vi "FT10_M4X Tester 2.vi"() -> ()   [LabVIEW 2024]
uses:
  Controls/QMH Fundamentals - Message Cluster.ctl
  <vilib>/FPGAPlugInAG/PXI-7854R/niLvFpga_Open_PXI-7854R.vi
  <vilib>/rvi/interface/common/dynamic/niFpgaDynamicAddResources.vi
  <vilib>/Utility/error.llb/Error Cluster From Error Code.vi
  <vilib>/rvi/errors/niLvFpgaAdjustHostInterfaceError.vi
  <vilib>/FPGAPlugInAG/Dynamic/niLvFpga_Close_Dynamic.vi
  <vilib>/rvi/interface/nirviOpenFPGA/nirviOpenFPGA.xnode
  FPGA Bitfiles/11_12_2024_FT10_FPGA_7854R_Main_Rev3 BitFile.lvbitx
  <vilib>/rvi/interface/nirviReadWriteControl/nirviReadWriteControl.xnode
  <vilib>/rvi/interface/nirviCloseFPGA/nirviCloseFPGA.xnode
  spcm_win32.dll
  NiFpgaLv.dll
  <vilib>/rvi/interface/Simulation/niFpgaSimulationCallBeginRW.vi
panel:
  in  "Conn2 - 75kHz":bool=TRUE
  in  "Conn2 - uSec Off":u16=6
  in  "Conn2 - uSec On":u16=7
  in  "Conn1/DIO_0_7 In":bool[](array[boolean])=[FALSE, FALSE, FALSE, FALSE, FALSE, FALSE, FALSE, FALSE]
  in  "Conn1/DIO_8_15 In":bool[](array[boolean])=[FALSE, FALSE, FALSE, FALSE, FALSE, FALSE, FALSE, FALSE]
  out "Conn1/DIO_0_7 Out":bool[](array[boolean])
  out "Conn1/DIO_8_15 Out":bool[](array[boolean])
  out "Conn1/DIO_16_23 Out":bool[](array[boolean])
  in  "Conn1/DIO_16_23 In":bool[](array[boolean])=[FALSE, FALSE, FALSE, FALSE, FALSE, FALSE, FALSE, FALSE]
  out "error out 2":errorcluster
  out "error out":errorcluster
  in  "Conn1 - uSec On":u16=7
  in  "Conn1 - uSec Off":u16=6
  in  "Conn1 - 75kHz":bool=TRUE
  in  "Conn2/DIO_0_7 In":bool[](array[boolean])=[FALSE, FALSE, FALSE, FALSE, FALSE, FALSE, FALSE, FALSE]
  in  "Conn2/DIO_8_15 In":bool[](array[boolean])=[FALSE, FALSE, FALSE, FALSE, FALSE, FALSE, FALSE, FALSE]
  out "Conn2/DIO_0_7 Out":bool[](array[boolean])
  out "Conn2/DIO_8_15 Out":bool[](array[boolean])
  out "Conn2/DIO_16_23 Out":bool[](array[boolean])
  in  "Conn2/DIO_16_23 In":bool[](array[boolean])=[FALSE, FALSE, FALSE, FALSE, FALSE, FALSE, FALSE, FALSE]
  out "Array":T1(array[cluster])
  out "Waveform Array":waveform(dbl)[](graph)
  in  "stop":bool
  in  "Read":bool
  # "Conn1/DIO_0_7"
  # "Conn1/DIO_8_15"
  # "Conn1/DIO_16_23"
  # "Conn2/DIO_0_7"
  # "Conn2/DIO_8_15"
  # "Conn2/DIO_16_23"
  # "INPUTS"
  # "OUTPUTS"
  # "INPUTS"
  # "OUTPUTS"
  # "INPUTS"
  # "OUTPUTS"
  # "INPUTS"
  # "OUTPUTS"
  # "INPUTS"
  # "OUTPUTS"
  # "INPUTS"
  # "OUTPUTS"
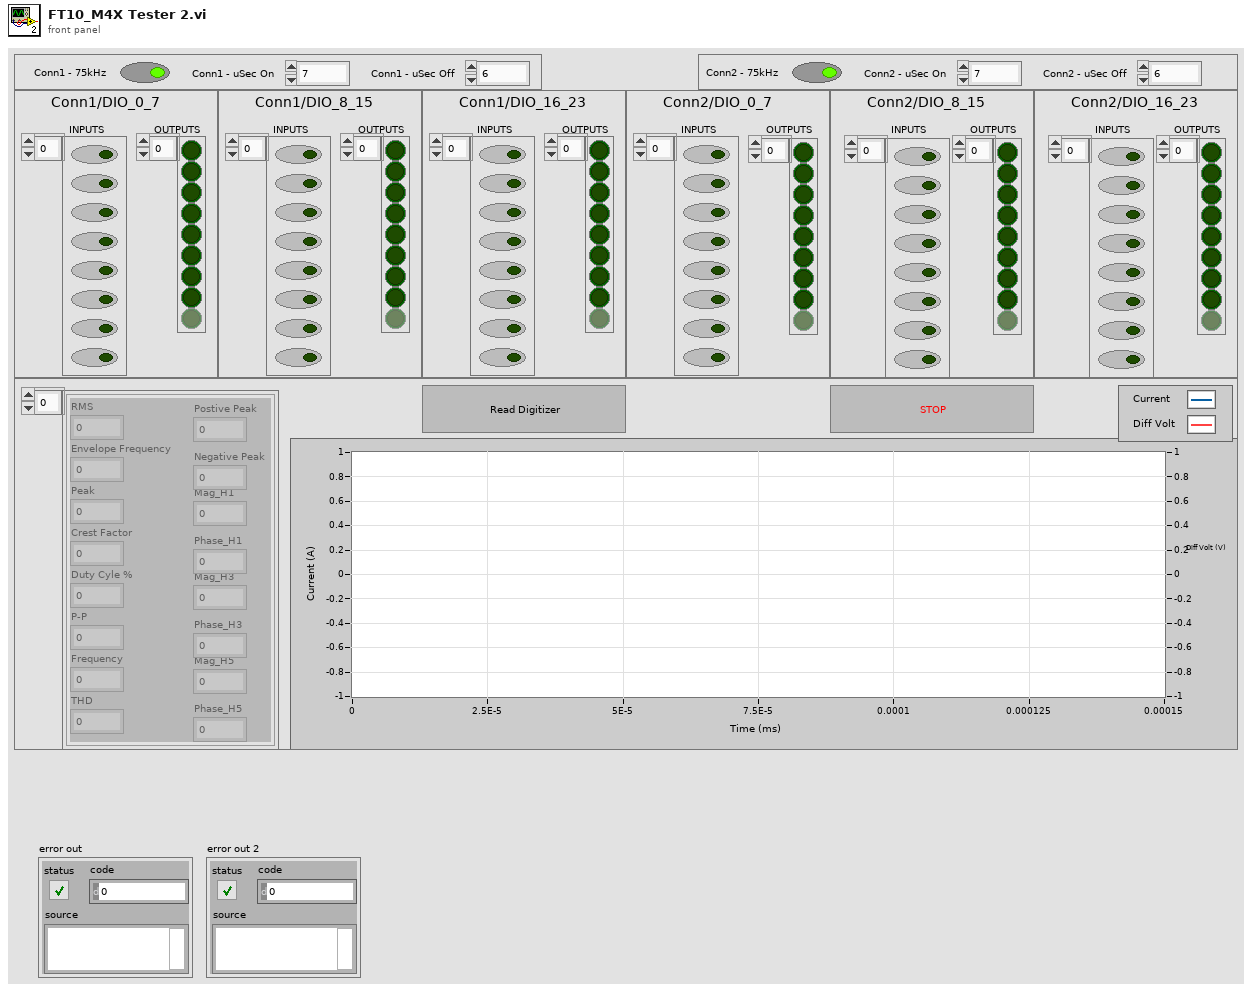
[diagram p1: front panel]
types:
  T1 = cluster{"RMS":dbl, "Envelope Frequency":dbl, "Peak":dbl, "Crest Factor":dbl, "Duty Cyle %":dbl, "P-P":dbl, "Frequency":dbl, "THD":dbl, "Postive Peak":dbl, "Negative Peak":dbl, "Mag_H1":dbl, "Phase_H1":dbl, "Mag_H3":dbl, "Phase_H3":dbl, "Mag_H5":dbl, "Phase_H5":dbl}[]
  T2 = typedef "QMH Fundamentals - Message Cluster.ctl" = cluster{"Message":string, "Message Data":variant}
  T3 = cluster{"RMS":dbl, "Envelope Frequency":dbl, "Peak":dbl, "Crest Factor":dbl, "Duty Cyle %":dbl, "P-P":dbl, "Frequency":dbl, "THD":dbl, "Postive Peak":dbl, "Negative Peak":dbl, "Mag_H1":dbl, "Phase_H1":dbl, "Mag_H3":dbl, "Phase_H3":dbl, "Mag_H5":dbl, "Phase_H5":dbl}
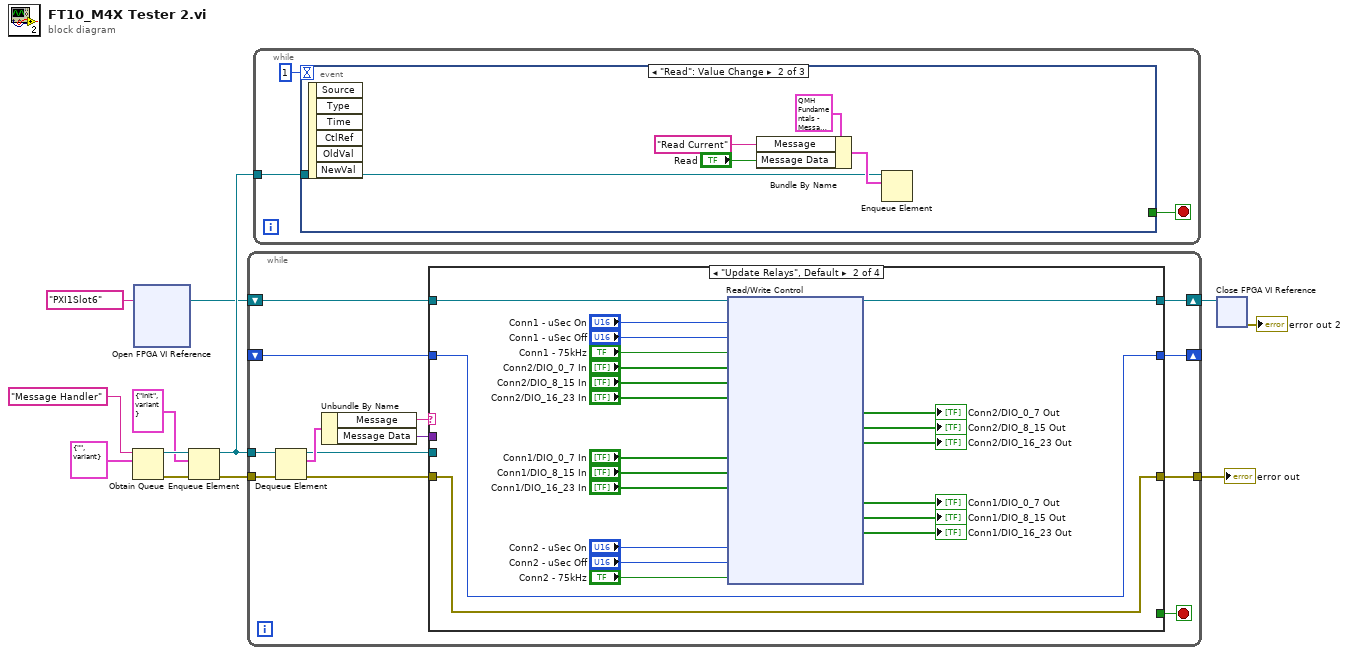
[diagram p0: block diagram]
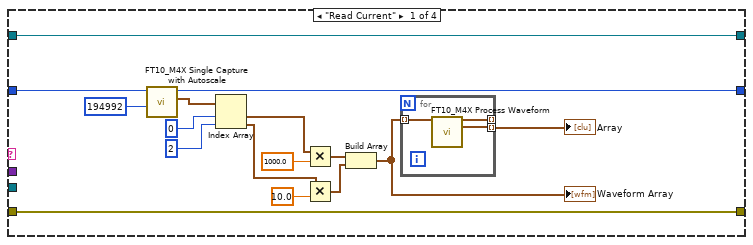
[diagram p2: hidden frame]
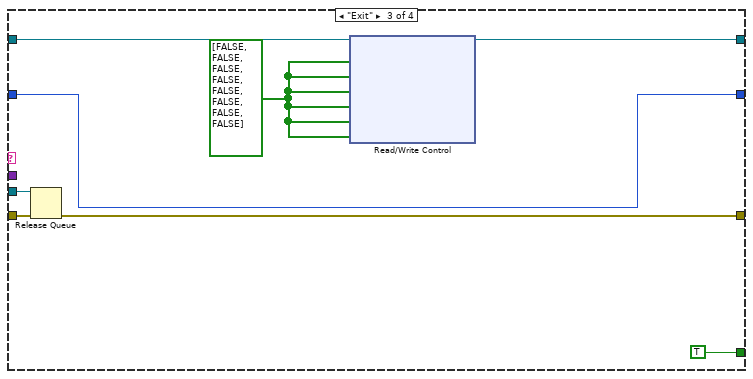
[diagram p3: hidden frame]
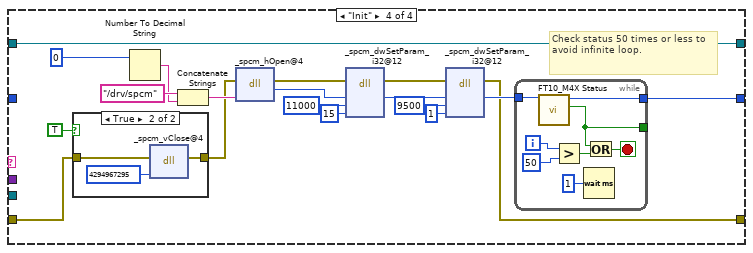
[diagram p4: hidden frame]
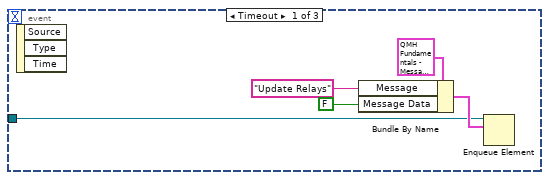
[diagram p6: hidden frame]
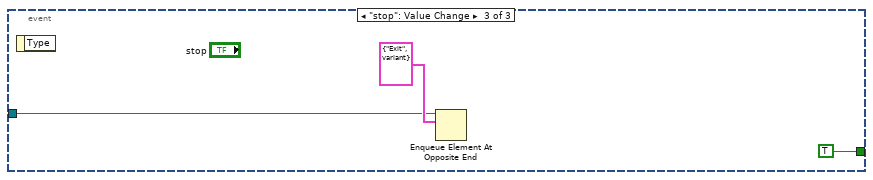
[diagram p7: hidden frame]
diagram:
  n1 = Obtain Queue(name (unnamed)="Message Handler", element data type=T2 {"Message"="", "Message Data"=variant} ("Message Cluster")) -> (queue out=w10:refnum<queue>, error out=w11:errorcluster)  [unwired: 3 in, 1 out]
  n2 = xnode "Open FPGA VI Reference"("resource name"=tag "PXI1Slot6") -> ("FPGA VI Reference Out"=w1:refnum<k20>)  [unwired: 1 in, 1 out]
  n3 = Enqueue Element(queue=w10, element=T2 {"Message"="Init", "Message Data"=variant}, error in (no error)=w11) -> (queue out=w5:refnum<queue>, error out=w7:errorcluster)  [unwired: 1 in, 1 out]
  n4 = while {
    tunnel: w5 -> [w24]
    tunnel: w7 -> [w23]
    tunnel: [w18] -> w6
    shift-right: [w17] -> _
    shift-left: _ -> [w16]
    shift-right: [w14] -> w4
    shift-left: w1 -> [w13]
    stop <- w15 stop-if-true
    n5 = Dequeue Element(queue=w24, error in (no error)=w23) -> (queue out=w22:refnum<queue>, element=w25:T2, error out=w21:errorcluster)  [unwired: 1 in, 1 out]
    n6 = Unbundle By Name(w25) -> ("Message"=w20:string, "Message Data"=w19:variant)
    n7 = case shown="\"Update Relays\", Default" w20 {
      tunnel: w22 -> [_ _ w71 _]
      tunnel: w21 -> [w30 w54 w73 w78]
      tunnel: w19 -> [_ _ _ _]
      tunnel: [w30 w54 w72 w77] -> w18
      tunnel: [w31 w55 w68 w76] -> w17
      tunnel: w16 -> [w32 w55 w68 _]
      tunnel: [_ _ TRUE _] -> w15
      tunnel: [w26 w56 w69 w75] -> w14
      tunnel: w13 -> [w26 w57 w70 w75]
      frame "Read Current" {
        n8 = call "FT10_M4X Single Capture with Autoscale.vi"("memsize"=194992, "Card Handle in"=w32) -> ("Data"=w35:waveform(sgl)[], "Card Handle out"=w31:u32)  [unwired: 8 in]
        n9 = Index Array(array=w35, index #1=0 ("index"), index #2=2 ("index 2")) -> (element #1=w40:waveform(sgl), element #2=w41:waveform(sgl))
        n10 = Multiply(x=w40, y=1000.0) -> (x*y=w38:waveform(dbl))
        n11 = Multiply(x=w41, y=10.0) -> (x*y=w39:waveform(dbl))
        n12 = Build Array(w38, w39) -> (w29:waveform(dbl)[])
        "Waveform Array" <- w29
        n13 = for {
          tunnel: w29 -> [w42] mode=indexing
          tunnel: [w44] -> w33 mode=indexing
          tunnel: [w43] -> _ mode=indexing
          n14 = call "FT10_M4X Process Waveform.vi"("RF Waveform In"=w42) -> ("RF Waveform Out"=w43:waveform(sgl), "Measurements"=w44:T3)  [unwired: 12 in, 1 out]
        }
        "Array" <- w33
      }
      frame "Update Relays", Default {
        n15 = xnode "Read/Write Control"("FPGA VI Reference In"=w57, "Conn1 - uSec On"="Conn1 - uSec On", "Conn1 - uSec Off"="Conn1 - uSec Off", "Conn1 - 75kHz"="Conn1 - 75kHz", "Conn2/DIO_0_7 In"="Conn2/DIO_0_7 In", "Conn2/DIO_8_15 In"="Conn2/DIO_8_15 In", "Conn2/DIO_16_23 In"="Conn2/DIO_16_23 In", "Conn1/DIO_0_7 In"="Conn1/DIO_0_7 In", "Conn1/DIO_8_15 In"="Conn1/DIO_8_15 In", "Conn1/DIO_16_23 In"="Conn1/DIO_16_23 In", "Conn2 - uSec On"="Conn2 - uSec On", "Conn2 - uSec Off"="Conn2 - uSec Off", "Conn2 - 75kHz"="Conn2 - 75kHz") -> ("FPGA VI Reference Out"=w56:refnum<k20>, "Conn2/DIO_0_7 Out"=→"Conn2/DIO_0_7 Out":bool[], "Conn2/DIO_8_15 Out"=→"Conn2/DIO_8_15 Out":bool[], "Conn2/DIO_16_23 Out"=→"Conn2/DIO_16_23 Out":bool[], "Conn1/DIO_0_7 Out"=→"Conn1/DIO_0_7 Out":bool[], "Conn1/DIO_8_15 Out"=→"Conn1/DIO_8_15 Out":bool[], "Conn1/DIO_16_23 Out"=→"Conn1/DIO_16_23 Out":bool[])  [unwired: 1 in, 1 out]
      }
      frame "Exit" {
        w67 = bool[] [FALSE, FALSE, FALSE, FALSE, FALSE, FALSE, FALSE, FALSE] ("Conn1/DIO_0_7 In")
        n16 = Release Queue(queue=w71, error in (no error)=w73) -> (error out=w72:errorcluster)  [unwired: 1 in, 2 out]
        n17 = xnode "Read/Write Control"("FPGA VI Reference In"=w70, "Conn1/DIO_0_7 In"=w67, "Conn1/DIO_8_15 In"=w67, "Conn1/DIO_16_23 In"=w67, "Conn2/DIO_0_7 In"=w67, "Conn2/DIO_8_15 In"=w67, "Conn2/DIO_16_23 In"=w67) -> ("FPGA VI Reference Out"=w69:refnum<k20>)  [unwired: 1 in, 1 out]
      }
      frame "Init" {
        # "Check status 50 times or less to avoid infinite loop."
        n18 = case shown="True" TRUE ("reset device") {
          tunnel: w78 -> [w102 w105]
          tunnel: [w102 w104] -> w88
          frame False {
          }
          frame True {
            n19 = dll-call lib="spcm_win32.dll" fn="_spcm_vClose@4"(error in=w105, "hDrv"=u32 4294967295) -> (error out=w104:errorcluster)  [unwired: 4 in, 1 out]
          }
        }
        n20 = Number To Decimal String(number=u32 0 ("Board #")) -> (decimal integer string=w89:string)  [unwired: 1 in]
        n21 = Concatenate Strings("/drv/spcm" ("szDeviceName"), w89) -> (w90:string)
        n22 = dll-call lib="spcm_win32.dll" fn="_spcm_hOpen@4"(error in=w88, "szDeviceName"=w90) -> (error out=w86:errorcluster, "hDrv"=w85:u32)  [unwired: 3 in, 1 out]
        n23 = dll-call lib="spcm_win32.dll" fn="_spcm_dwSetParam_i32@12" label="SPC_CHENABLE"(error in=w86, "hDrv"=w85, "lRegister"=11000, "lValue"=15) -> (error out=w82:errorcluster, "hDrv"=w81:u32)  [unwired: 5 in, 1 out]
        n24 = dll-call lib="spcm_win32.dll" fn="_spcm_dwSetParam_i32@12" label="SPC_CARDMODE"(error in=w82, "hDrv"=w81, "lRegister"=9500, "lValue"=1) -> (error out=w77:errorcluster, "hDrv"=w93:u32)  [unwired: 5 in, 1 out]
        n25 = while {
          tunnel: w93 -> [w100]
          tunnel: [w99] -> w76
          tunnel: [w94] -> _
          i -> [w98]
          stop <- w96 stop-if-true
          n26 = call "FT10_M4X Status.vi"("Card Handle in"=w100) -> ("Ready?"=w94:bool, "Card Handle out"=w99:u32)  [unwired: 9 in]
          n27 = Greater?(x=w98, y=50) -> (0:w95:bool)
          n28 = Wait (ms)(milliseconds to wait=u32 1) -> ()  [unwired: 1 out]
          n29 = Or(x=w94, y=w95) -> (x .or. y?=w96:bool)
        }
      }
    }
  }
  "error out" <- w6
  n30 = while {
    tunnel: w5 -> [w108]
    stop <- w107 stop-if-true
    n31 = event shown="[1] \"Read\": Value Change" {
      selector: _ -> [_ _ _]
      dyn-events: _ -> [_ _ _]
      timeout: 1 -> [_ _ _]
      tunnel: w108 -> [w109 w115 w120]
      tunnel: [_ _ TRUE] -> w107
      event Timeout {
        n32 = event-data() -> ()  [unwired: 1 in, 3 out]
        n33 = Bundle By Name(cluster=T2 {"Message"="Fornax Connect/Disconnect", "Message Data"=variant} ("element"), "Message"="Update Relays", "Message Data"=FALSE ("Update Relays 2")) -> (w111:T2)
        n34 = Enqueue Element(queue=w109, element=w111) -> ()  [unwired: 2 in, 3 out]
      }
      event "Read": Value Change {
        n35 = event-data() -> ()  [unwired: 1 in, 6 out]
        n36 = Bundle By Name(cluster=T2 {"Message"="Fornax Connect/Disconnect", "Message Data"=variant} ("element"), "Message"="Read Current", "Message Data"="Read") -> (w116:T2)
        n37 = Enqueue Element(queue=w115, element=w116) -> ()  [unwired: 2 in, 3 out]
      }
      event "stop": Value Change {
        n38 = event-data() -> ()  [unwired: 1 in, 1 out]
        n39 = Enqueue Element At Opposite End(queue=w120, element=T2 {"Message"="Exit", "Message Data"=variant}) -> ()  [unwired: 2 in, 3 out]
      }
    }
  }
  n40 = xnode "Close FPGA VI Reference"("FPGA VI Reference In"=w4) -> ("error out"=→"error out 2":errorcluster)  [unwired: 1 in]
